vi "5.vi"() -> ()   [LabVIEW 2017]
uses:
  <userlib>/_OpenG.lib/string/string.llb/Convert EOLs (String)__ogtk.vi
  <userlib>/_OpenG.lib/string/string.llb/Trim Whitespace (String Array)__ogtk.vi
  <userlib>/_OpenG.lib/array/array.llb/Filter 1D Array with Scalar (String)__ogtk.vi
panel:
  out "delimited string":string
  out "filtered array":string[](array[string])
  out "Array":dbl[](array[numeric])
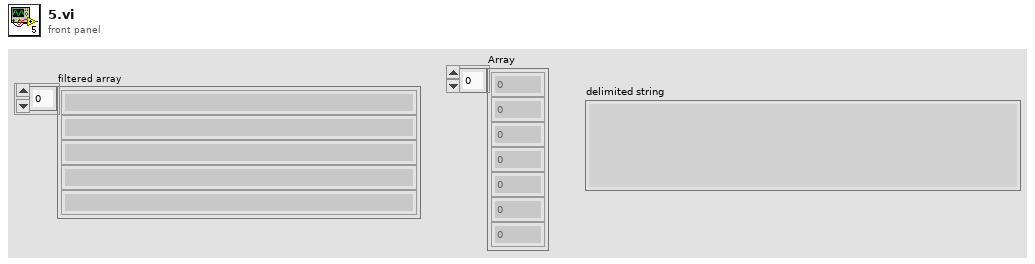
[diagram p1: front panel]
types:
  T1 = enum16{"open", "replace", "create", "open or create", "replace or create", "replace or create with confirmation"}
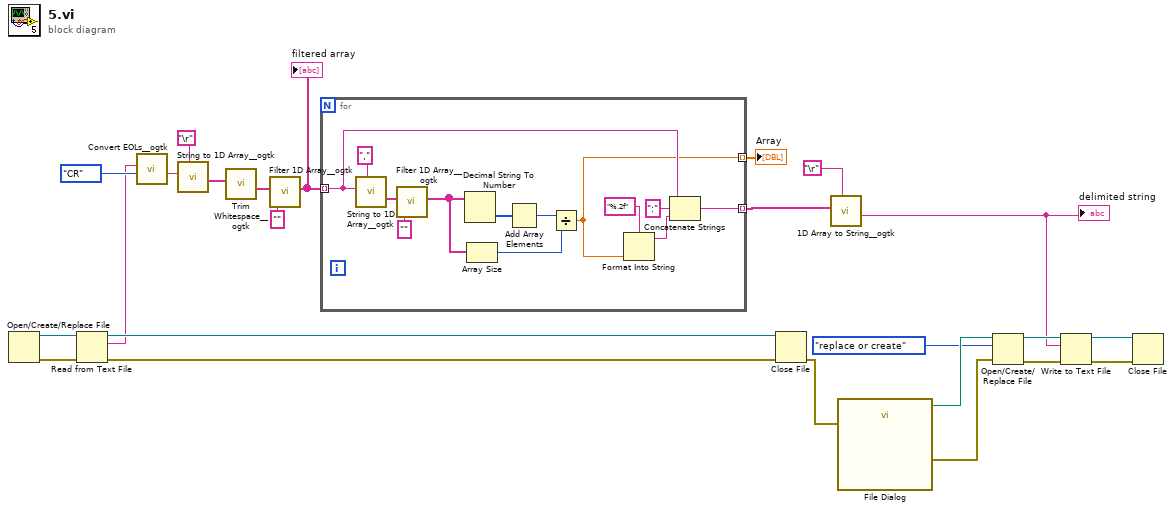
[diagram p0: block diagram]
diagram:
  n1 = Open/Create/Replace File() -> (refnum out=w24:refnum<file>, error out=w23:errorcluster)  [unwired: 6 in, 1 out]
  n2 = Read from Text File(file (use dialog)=w24, error in=w23) -> (refnum out=w22:refnum<file>, text=w19:string, error out=w21:errorcluster)  [unwired: 2 in, 1 out]
  n3 = call-poly <userlib>:"Convert EOLs__ogtk.vi"("Convert to:"=enum16{"CR", "LF", "CRLF"}."CR", "String in"=w19) -> ("String out"=w18:string)  [unwired: 9 in]
  n4 = call <userlib>:"String to 1D Array__ogtk.vi"("delimiter (Tab)"="\r", "string"=w18) -> ("Array of Strings"=w16:string[])  [unwired: 9 in]
  n5 = call-poly <userlib>:"Trim Whitespace__ogtk.vi"("String in"=w16) -> ("String out"=w15:string[])  [unwired: 6 in]
  n6 = call-poly <userlib>:"Filter 1D Array__ogtk.vi"("items to filter"="" ("delimiter (Tab)"), "array"=w15) -> ("filtered array"=w13:string[])  [unwired: 4 in, 1 out]
  "filtered array" <- w13
  n7 = for {
    tunnel: w13 -> [w30] mode=indexing
    tunnel: [w28] -> w8 mode=indexing
    tunnel: [w25] -> w7 mode=indexing
    n8 = call <userlib>:"String to 1D Array__ogtk.vi"("delimiter (Tab)"=",", "string"=w30) -> ("Array of Strings"=w35:string[])  [unwired: 9 in]
    n9 = call-poly <userlib>:"Filter 1D Array__ogtk.vi"("items to filter"="" ("delimiter (Tab)"), "array"=w35) -> ("filtered array"=w32:string[])  [unwired: 4 in, 1 out]
    n10 = Decimal String To Number(string=w32) -> (number=w34:i32[])  [unwired: 2 in, 1 out]
    n11 = Array Size(array=w32) -> (size(s)=w31:i32)
    n12 = Add Array Elements(numeric array=w34) -> (sum=w33:i32)
    n13 = Divide(x=w33, y=w31) -> (x/y=w28:dbl)
    n14 = Format Into String(format string="%.2f", w28) -> (resulting string=w27:string)  [unwired: 2 in, 1 out]
    n15 = Concatenate Strings(w30, ":" ("string"), w27) -> (w25:string)
  }
  "Array" <- w8
  n16 = Close File(refnum=w22, error in=w21) -> (error out=w2:errorcluster)  [unwired: 1 out]
  n17 = call <userlib>:"1D Array to String__ogtk.vi"("delimiter (Tab)"="\r", "Array of Strings"=w7) -> ("delimited string"=w5:string)  [unwired: 9 in]
  "delimited string" <- w5
  n18 = call "File Dialog"("error in"=w2) -> ("selected path"=w4:path, "error out"=w3:errorcluster)  [unwired: 11 in, 2 out]
  n19 = Open/Create/Replace File(file path (use dialog)=w4, error in=w3, operation (0:open)=T1."replace or create") -> (refnum out=w9:refnum<file>, error out=w10:errorcluster)  [unwired: 3 in, 1 out]
  n20 = Write to Text File(file (use dialog)=w9, text=w5, error in=w10) -> (refnum out=w11:refnum<file>, error out=w12:errorcluster)  [unwired: 1 in, 1 out]
  n21 = Close File(refnum=w11, error in=w12) -> ()  [unwired: 2 out]
